vi "Picture properties.vi"() -> ()   [LabVIEW 2009]
uses:
  object.ctl
  <vilib>/Utility/miscctls.llb/LVPositionTypeDef.ctl
panel:
  in  "stop":bool
  in  "clear picture":bool
  in  "value":dbl(slide) scale=-10.0..10.0
  out "Pic":picture
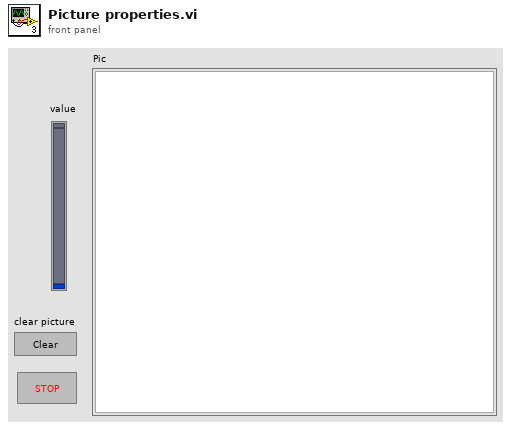
[diagram p1: front panel]
types:
  T1 = typedef "LVPositionTypeDef.ctl" = cluster{"Left":i32, "Top":i32}
  T2 = typedef "object.ctl" = cluster{"rect":cluster{"left":i16, "top":i16, "right":i16, "bottom":i16}, "weight":sgl}
  T3 = cluster{"left":i16, "top":i16, "right":i16, "bottom":i16}
  T4 = typedef "LVPoint32TypeDef.ctl" = cluster{"Horizontal":i32, "Vertical":i32}
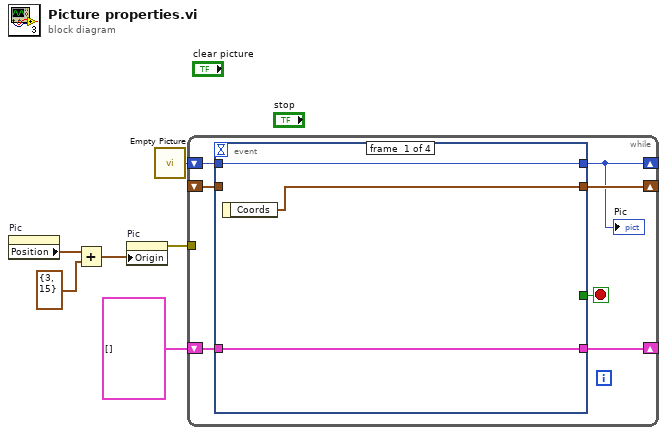
[diagram p0: block diagram]
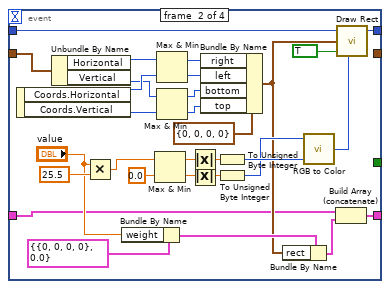
[diagram p2: hidden frame]
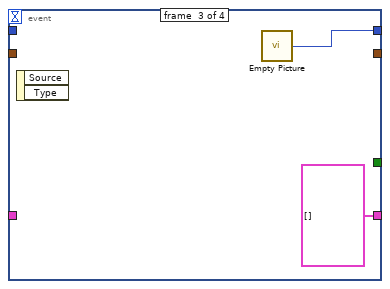
[diagram p3: hidden frame]
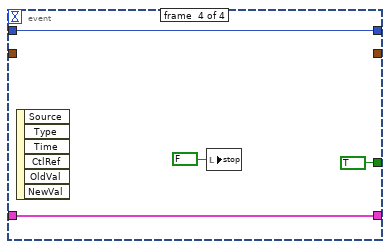
[diagram p4: hidden frame]
diagram:
  n1 = property on="Pic" class="Pict"() -> ("Position"=w3:T1)  [unwired: 2 in, 2 out]
  n2 = Add(x=w3, y=T1 {"Left"=3, "Top"=15}) -> (x+y=w1:T1)
  n3 = property on="Pic" class="Pict"("Origin"=w1) -> (error out=w4:errorcluster)  [unwired: 2 in, 1 out]
  n4 = call "Empty Picture"() -> ("empty picture"=w5:picture)
  n5 = while {
    shift-right: [w13] -> _
    shift-left: _ -> [w12]
    shift-right: [w7] -> _
    shift-left: w5 -> [w11]
    shift-right: [w8] -> _
    shift-left: T2[] [] -> [w9]
    tunnel: w4 -> [_]
    stop <- w10 stop-if-true
    n6 = event shown="[1] \"Pic\": Mouse Up" {
      selector: _ -> [_ _ _ _]
      dyn-events: _ -> [_ _ _ _]
      timeout: _ -> [_ _ _ _]
      tunnel: [w16 _ _ _] -> w13
      tunnel: w12 -> [_ w46 _ _]
      tunnel: [w15 w41 w47 w50] -> w7
      tunnel: w11 -> [w15 w40 _ w50]
      tunnel: [_ _ _ TRUE] -> w10
      tunnel: w9 -> [w14 w17 _ w51]
      tunnel: [w14 w18 T2[] [] w51] -> w8
      event #0 {
        n7 = event-data() -> ("Coords"=w16:T4)  [unwired: 1 in]
      }
      event #1 {
        n8 = event-data() -> ("Coords.Horizontal"=w44:i32, "Coords.Vertical"=w42:i32)  [unwired: 1 in]
        n9 = Unbundle By Name(w46) -> ("Horizontal"=w45:i32, "Vertical"=w43:i32)
        n10 = Multiply(x="value", y=25.5) -> (x*y=w32:dbl)
        n11 = Bundle By Name(cluster=T2 {"rect"={"left"=0, "top"=0, "right"=0, "bottom"=0}, "weight"=0.0} ("Object"), "weight"="value") -> (w21:T2)
        n12 = Max & Min(x=w32, y=0.0) -> (max(x,y)=w30:dbl, min(x,y)=w29:dbl)
        n13 = Max & Min(x=w45, y=w44) -> (max(x,y)=w35:i32, min(x,y)=w36:i32)
        n14 = Max & Min(x=w43, y=w42) -> (max(x,y)=w38:i32, min(x,y)=w37:i32)
        n15 = Absolute Value(x=w30) -> (abs(x)=w28:dbl)
        n16 = Absolute Value(x=w29) -> (abs(x)=w27:dbl)
        n17 = Bundle By Name(cluster=T3 {"left"=0, "top"=0, "right"=0, "bottom"=0} ("rect"), "right"=w35, "left"=w36, "bottom"=w38, "top"=w37) -> (w20:T3)
        n18 = To Unsigned Byte Integer(number=w28) -> (unsigned 8bit integer=w26:u8)
        n19 = To Unsigned Byte Integer(number=w27) -> (unsigned 8bit integer=w25:u8)
        n20 = Bundle By Name(cluster=w21, "rect"=w20) -> (w19:T2)
        n21 = call <vilib>:"RGB to Color.vi"("B"=w26, "R"=w25) -> ("Color"=w24:u32)  [unwired: 1 in]
        n22 = Build Array (concatenate)(w17, w19) -> (w18:T2[])
        n23 = call <vilib>:"Draw Rect.vi"("picture"=w40, "rect"=w20, "fill?(F)"=TRUE, "color(black)"=w24) -> ("new picture"=w41:picture)  [unwired: 5 in]
      }
      event #2 {
        n24 = event-data() -> ()  [unwired: 1 in, 2 out]
        n25 = call "Empty Picture"() -> ("empty picture"=w47:picture)
      }
      event #3 {
        n26 = event-data() -> ()  [unwired: 1 in, 6 out]
        n27 = local write "stop"(FALSE ("stop")) -> ()
      }
    }
    "Pic" <- w7
  }
